vi "Get Thread Configuration.vi"(8 "error in (no error)":errorcluster, 11 "Component Configuration in":refnum<class "UDPlog Configurations.lvclass">) -> (0 "error out":errorcluster, 2 "Thread Configuration":refnum<class "Configuration.lvclass">, 3 "Component Configuration out":refnum<class "UDPlog Configurations.lvclass">)   [LabVIEW 2023, in "UDPlog.lvlib" / "UDPlog Configurations.lvclass"]
uses:
  UDPlog Configurations.lvclass
  UDPlog Configurations.lvclass/UDPlog Configurations.ctl
  Thread/UDPlog Thread Configuration.lvclass
  C:/Program Files/National Instruments/LabVIEW 2023/Vi.Lib/AddOns/VeriStand Custom Device Scripting APIs/Data Sharing Framework/DSF Core.lvlibp/Classes/Configuration/Configuration.lvclass
  C:/git/niveristand-data-sharing-framework-custom-device-plugins/Components/Transceivers/UDPlog/Source/Configurations/Thread/UDPlog Thread Configuration.lvclass
  <vilib>/AddOns/VeriStand Custom Device Scripting APIs/Data Sharing Framework/DSF Core.lvlibp/Classes/Configuration/Configuration.lvclass
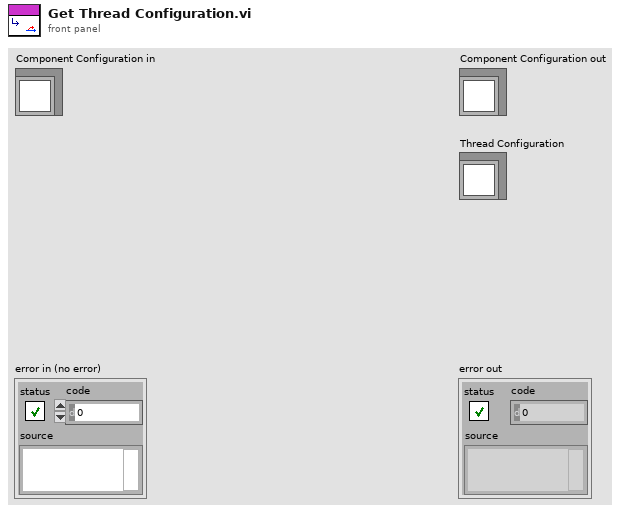
[diagram p1: front panel]
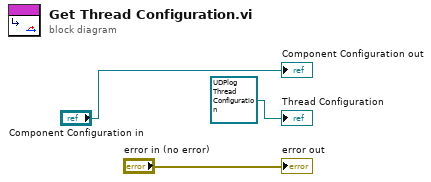
[diagram p0: block diagram]
diagram:
  "error out" <- "error in (no error)"
  "Component Configuration out" <- "Component Configuration in"
  "Thread Configuration" <- refnum<class "UDPlog Thread Configuration.lvclass"> refnum ("UDPlog.lvlib:UDPlog Thread Configuration.lvclass")
